vi "from_string.vi"(8 "error in (no error)":errorcluster, 10 "toml":string) -> (0 "error out":errorcluster, 3 "toml out":refnum<class "toml.lvclass">)   [LabVIEW 2020, in "toml.lvclass"]
uses:
  toml.lvclass
  toml.lvclass/toml.ctl
  Doc/Doc.lvclass
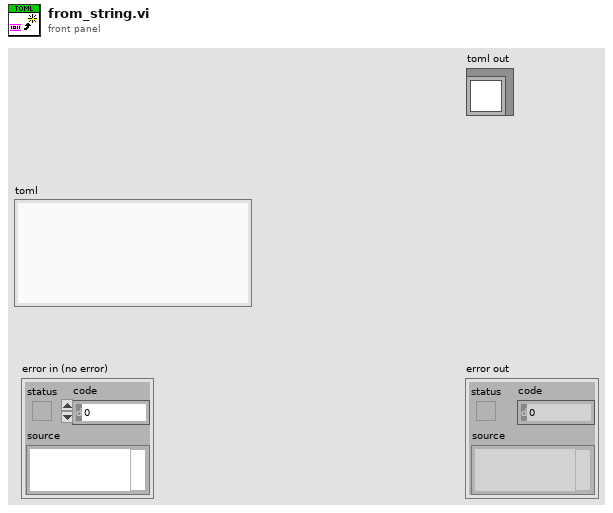
[diagram p1: front panel]
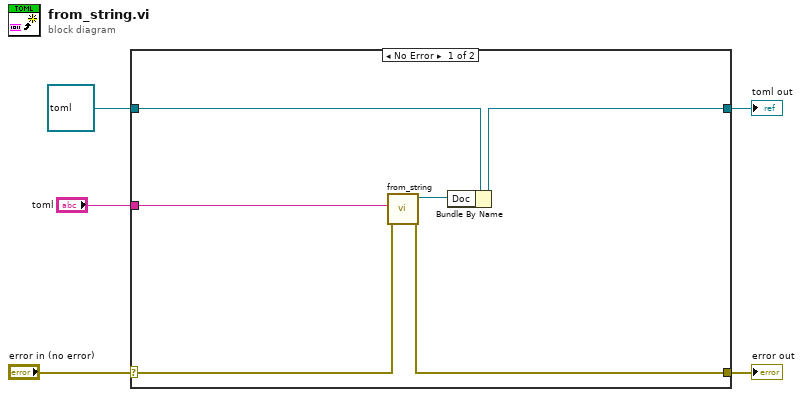
[diagram p0: block diagram]
diagram:
  n1 = case shown="No Error" "error in (no error)" {
    selector: "error in (no error)" -> [w7 w13]
    tunnel: [w6 w13] -> w4
    tunnel: [w9 w12] -> w2
    tunnel: refnum<class "toml.lvclass"> refnum ("toml in") -> [w11 w12]
    tunnel: "toml" -> [w10 _]
    frame No Error {
      n2 = call "from_string.vi"("error in (no error)"=w7, "toml"=w10) -> ("error out"=w6:errorcluster, "Doc out"=w8:refnum<class "Doc.lvclass">)  [unwired: 8 in]
      n3 = Bundle By Name(cluster=w11, "Doc"=w8) -> (w9:refnum<class "toml.lvclass">)
    }
    frame Error {
    }
  }
  "error out" <- w4
  "toml out" <- w2
